vi "Arb ID to Unique Name.vi"(11 "Arb ID":u32 format="%.0x") -> (3 "name":string)   [LabVIEW 2013, in "J1939.lvlib"]
uses:
  J1939.lvlib
  Frame Conversion/Convert CAN Arb ID to J1939 ID.vi
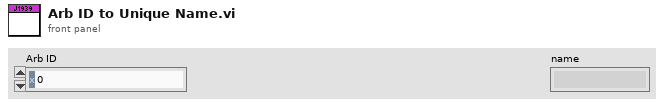
[diagram p1: front panel]
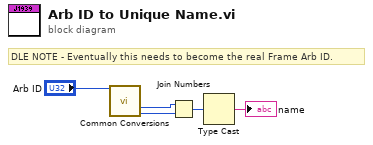
[diagram p0: block diagram]
diagram:
  # "DLE NOTE - Eventually this needs to become the real Frame Arb ID."
  n1 = call-poly "Common Conversions.vi"("Arb ID"="Arb ID") -> ("PGN"=w4:u32, "Source Address"=w5:u8)  [unwired: 13 out]
  n2 = Join Numbers(hi=w4, lo=w5) -> ((hi.lo)=w3:u64)
  n3 = Type Cast(x=w3) -> (*(type *) &x=→"name":string)  [unwired: 1 in]
